vi "open motor.vi"(8 "error in":errorcluster, 11 "COM port":string) -> (0 "error out":errorcluster, 2 "Motor ID":string, 3 "CONEX_CC":refnum<k24>)   [LabVIEW 2017]
uses:
  Newport.CONEXCC.CommandInterface
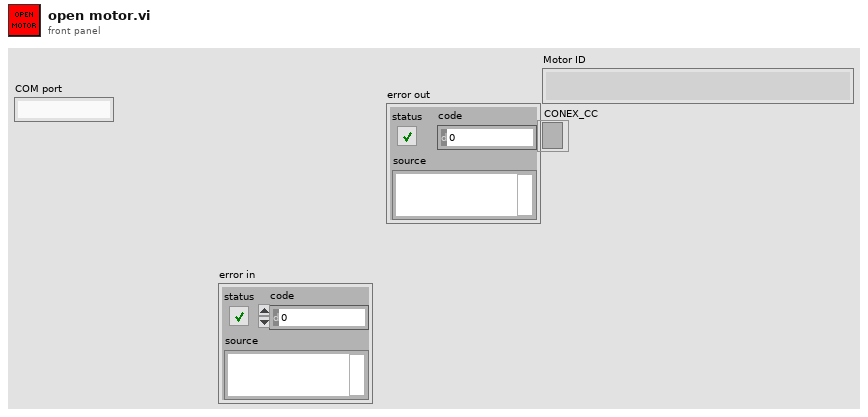
[diagram p1: front panel]
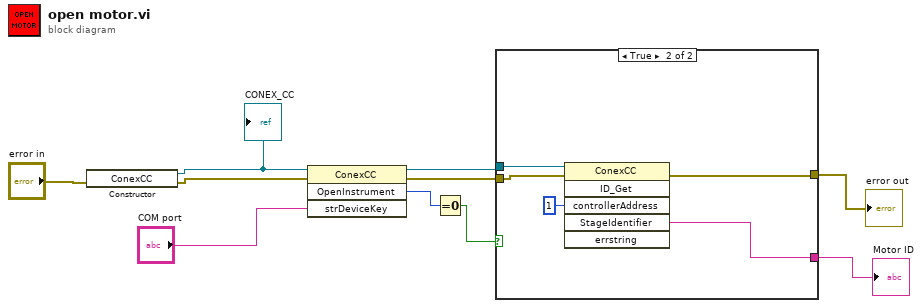
[diagram p0: block diagram]
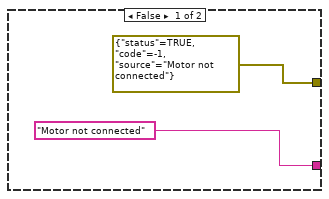
[diagram p2: hidden frame]
diagram:
  n1 = constructor class="ConexCC"(error in="error in") -> (reference out=w10:refnum<k24>, error out=w1:errorcluster)  [unwired: 2 in, 1 out]
  "CONEX_CC" <- w10
  n2 = invoke class="ConexCC" method="OpenInstrument"(reference=w10, error in=w1, "strDeviceKey"="COM port") -> (reference out=w4:refnum<k24>, error out=w7:errorcluster, "OpenInstrument"=w8:i32)  [unwired: 1 in, 1 out]
  n3 = Equal To 0?(x=w8) -> (x = 0?=w6:bool)
  n4 = case shown="True" w6 {
    tunnel: w4 -> [_ w15]
    tunnel: w7 -> [_ w16]
    tunnel: [errorcluster {"status"=TRUE, "code"=-1, "source"="Motor not connected"} ("error constant") w13] -> w5
    tunnel: ["Motor not connected" ("StageIdentifier") w14] -> w3
    frame False {
    }
    frame True {
      n5 = invoke class="ConexCC" method="ID_Get"(reference=w15, error in=w16, "controllerAddress"=1) -> (error out=w13:errorcluster, "StageIdentifier"=w14:string)  [unwired: 3 in, 4 out]
    }
  }
  "error out" <- w5
  "Motor ID" <- w3
